vi "Main.vi"() -> ()   [LabVIEW 2025]
panel:
  out "Acceleration Z":i16
  out "Acceleration Y":i16
  in  "stop":bool
  out "Acceleration X":i16
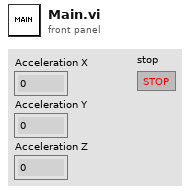
[diagram p1: front panel]
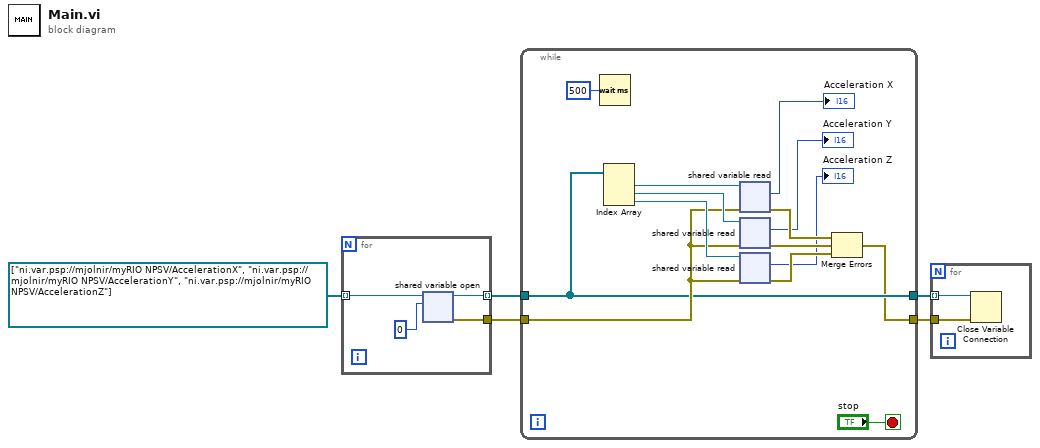
[diagram p0: block diagram]
diagram:
  n1 = for {
    tunnel: [w9] -> w5 mode=indexing
    tunnel: [w8] -> w4
    tunnel: refnum<k21>[] ["ni.var.psp://mjolnir/myRIO NPSV/AccelerationX", "ni.var.psp://mjolnir/myRIO NPSV/AccelerationY", "ni.var.psp://mjolnir/myRIO NPSV/AccelerationZ"] -> [w6] mode=indexing
    n2 = shared-variable-open(w6, i16 0) -> (w9:refnum<k21>, w8:errorcluster)  [unwired: 2 in]
  }
  n3 = while {
    tunnel: w5 -> [w16]
    tunnel: [w16] -> w1
    tunnel: w4 -> [w17]
    tunnel: [w15] -> w2
    stop <- "stop" stop-if-true
    n4 = Wait (ms)(milliseconds to wait=u32 500) -> ()  [unwired: 1 out]
    n5 = Index Array(array=w16) -> (element #1=w20:refnum<k21>, element #2=w19:refnum<k21>, element #3=w18:refnum<k21>)  [unwired: 3 in]
    n6 = shared-variable-read(w20, w17) -> (w14:errorcluster, →"Acceleration X":i16)  [unwired: 2 out]
    n7 = shared-variable-read(w19, w17) -> (w13:errorcluster, →"Acceleration Y":i16)  [unwired: 2 out]
    n8 = shared-variable-read(w18, w17) -> (w12:errorcluster, →"Acceleration Z":i16)  [unwired: 2 out]
    n9 = Merge Errors(w14, w13, w12) -> (w15:errorcluster)
  }
  n10 = for {
    tunnel: w2 -> [w25]
    tunnel: w1 -> [w24] mode=indexing
    n11 = Close Variable Connection(8:w25, 11:w24) -> ()  [unwired: 1 out]
  }
